vi "Alarmnum variable.vi"() -> ()   [LabVIEW 2010]
panel:
  in  "# of Alarms":i16
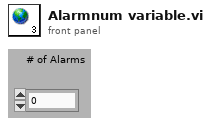
[diagram p1: front panel]
diagram:
